vi "Project selector.vi"(11 "error in (no error)":errorcluster) -> (8 "OK":bool, 15 "error out":errorcluster)   [LabVIEW 2011]
doc: "Welcome screen, with basic options"
uses:
  GUI/Job setup/Job and site cluster.ctl
  emi cndiates/List of all contrys(combo box).ctl
  GUI/Job setup/Tool registration ID.ctl
  GUI/Job setup/Operators display clustor.ctl
  Application Structure/User Control/User Indikator.ctl
  Application Structure/User Control/Super User bool indikator.ctl
  Project infor with project path.ctl
  Project in icluster.ctl
  Run Information.ctl
panel:
  out "Comment":string
  in  "Project selector":u16(ring) items=["4325", "789"]
  in  "New project":bool
  in  "Operators":T1
  out "Tool":T2
  out "Job & Site":T3
  in  "Cancel":bool
  in  "OK btn":bool
  # "Comment"
  # "Tab header s can be changed as wanted\n\nCustom can be used for completly ccutom behavior,\nmust then highjack  an other hidden page, for settings"
  # "Add custom behavior taht cvan not be replicated by a simple cluster with valisdity checking"
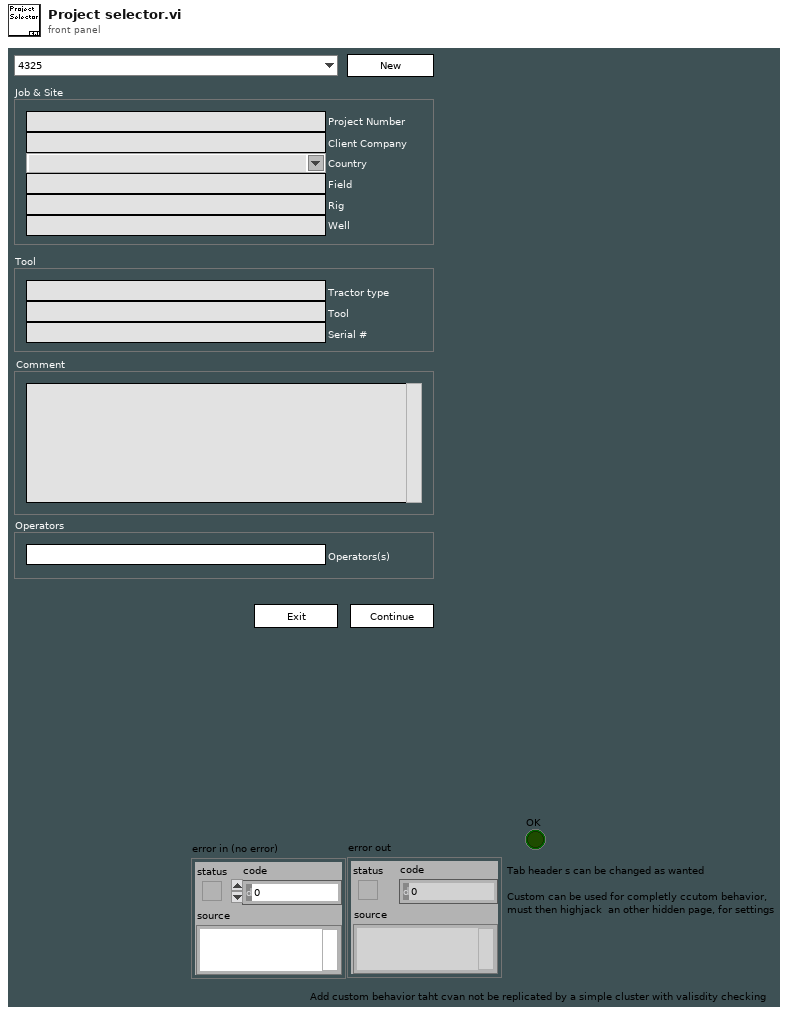
[diagram p1: front panel]
types:
  T1 = typedef "Operators display clustor.ctl" = cluster{"Operators(s)":string}
  T2 = typedef "Tool registration ID.ctl" = cluster{"Tractor type":string, "Tool":string, "Serial #":string}
  T3 = typedef "Job and site cluster.ctl" = cluster{"Project Number":string, "Client Company":string, "Country":T4, "Field":string, "Rig":string, "Well":string}
  T4 = typedef "List of all contrys(combo box).ctl" = string
  T5 = enum16{"GET", "SET", "Get from Ini", "Put in Ini"}
  T6 = typedef "User Indikator.ctl" = cluster{"User Name":string, "Super User":T7}
  T7 = typedef "Super User bool indikator.ctl" = bool
  T8 = typedef "Options  All pages and custom.ctl" = cluster{"P 1 (App)":T9, "P 2":T10, "P 3":T11, "P 4":T14, "P 5":T19, "P 6 (Err)":T20, "P 7 (Expert)":T21, "P 8 (Depth)":T23, "C 1":T24, "C 2":T25}
  T9 = typedef "Options Page 1 (App).ctl" = cluster{"Result files":path, "PCP Interface":string, "Tractor/Stroker Interface":string, "Tractor Interface":string, "Modem Status Interface":string, "Audible Alarm":bool, "Force alarm on Technical":bool, "Force alarm on HH":bool, "Force alarm on LL":bool, "Force alarm on H":bool, "Force alarm on L":bool}
  T10 = typedef "Options Page 2.ctl" = cluster{"Solenoid & Relay latching time":u16, "Tractor relay 1":dbl, "Tractor relay 2":dbl, "Tractor Solenoid limit":dbl}
  T11 = typedef "Options Page 3.ctl" = cluster{"Min resistance":dbl, "Max resistance":dbl, "Head voltage range":T12, "Max voltage jump":dbl, "Maximum resistance change":dbl, "Start Telemetry Voltage":dbl, "Start Telemetry Timeout":dbl, "Start Motor Voltage":dbl, "Stop Motor Voltage":dbl, "Pass Mode Warning Voltage":dbl, "Relay Switch Voltage":dbl, "Relay Status Loss Voltage":dbl, "Samples to average":i32, "PSU type DO NOT USE":T13, "Magna OVP":dbl, "Magna Current Limit":dbl}
  T12 = typedef "PCP type List.ctl" = enum16{"0 - 350V", "0 - 450V", "0 - 600V"}
  T13 = typedef "PSU Type.ctl" = enum16{"Unipower", "Magna 8.3A", "Magna 12A", "None"}
  T14 = typedef "Options Page 4.ctl" = cluster{"Solenoid & Relay latching time":u16, "Stroker relay 1":dbl, "Stroker Relay 2":dbl, "Stroker Solenoid limit":dbl, "Force det.":T15, "Stroke force lim.":dbl, "Anchor Enabled Pressure":dbl, "Tacometer puls":dbl, "Default anchor behavior":T16, "Default stroker behavior":T17, "Default stroker force limit (tonne)":dbl, "Slips Size":T18}
  T15 = typedef "Stroke force selector.ctl" = enum16{"Stroke in = node 1", "Strok out = node 1"}
  T16 = typedef "Default anchor behavior.ctl" = enum16{"Do nothing", "Set Anchor", "Release Anchor"}
  T17 = typedef "Default stroker behavior.ctl" = enum16{"Do nothing", "Stop", "Go Out", "Go In"}
  T18 = typedef "Slips Type Radio.ctl" = enum32{"No Selection", "338 MRS", "3,9 MRS"}
  T19 = typedef "Options Page 5.ctl" = cluster{"Solenoid & Relay latching time":u16, "Driller relay 1":dbl, "Driller Relay 2":dbl, "Driller  Solenoid limit":dbl}
  T20 = typedef "Options Page 6 (Err).ctl" = cluster{"Error and event files":path}
  T21 = typedef "Options Page 7 (Expert).ctl" = cluster{"Show Debug":bool, "Log debug messages":bool, "Additional debug messages":bool, "Start Beagle with Simulator data":bool, "Workshop mode":bool, "Modem baud":u16, "enumCANCOM":bool, "Modem sim":T22, "Telemetry Timeout Disable":i32, "Buffer size":i32, "Upd regular data":bool, "Cable comp":cluster{"VMOD1 Voltage(V)":dbl, "VMOD2 Voltage(V)":dbl}}
  T22 = typedef "Modem simulation setup.ctl" = cluster{"Modem dealay sim":bool, "Sim baud Tx":u16, "Bit Error fraction Tx":dbl, "Sim baud Rx":u16, "Bit Error fraction Rx":dbl}
  T23 = typedef "Options Page 8 (Depth).ctl" = cluster{"Winch Spool Circumference":dbl, "Winch Pulses per Revolution":dbl, "Current Depth":dbl}
  T24 = typedef "Options Custom 1.ctl" = cluster{"Depth Updated":bool, "Depth Offset":dbl}
  T25 = typedef "Options Custom 2.ctl" = cluster{"Placeholder":bool}
  T26 = typedef "Project infor with project path.ctl" = cluster{"Project path":path, "data":T27, "Comment":string}
  T27 = typedef "Project in icluster.ctl" = cluster{"Job and Site":T3, "Tool":T2, "Run Information":T28}
  T28 = typedef "Run Information.ctl" = cluster{"Active Run":bool, "String Check Rec":bool, "Run Number":i32, "Time of File Start":string}
  T29 = enum8{"Enabled", "Disabled", "Disabled and Grayed Out"}
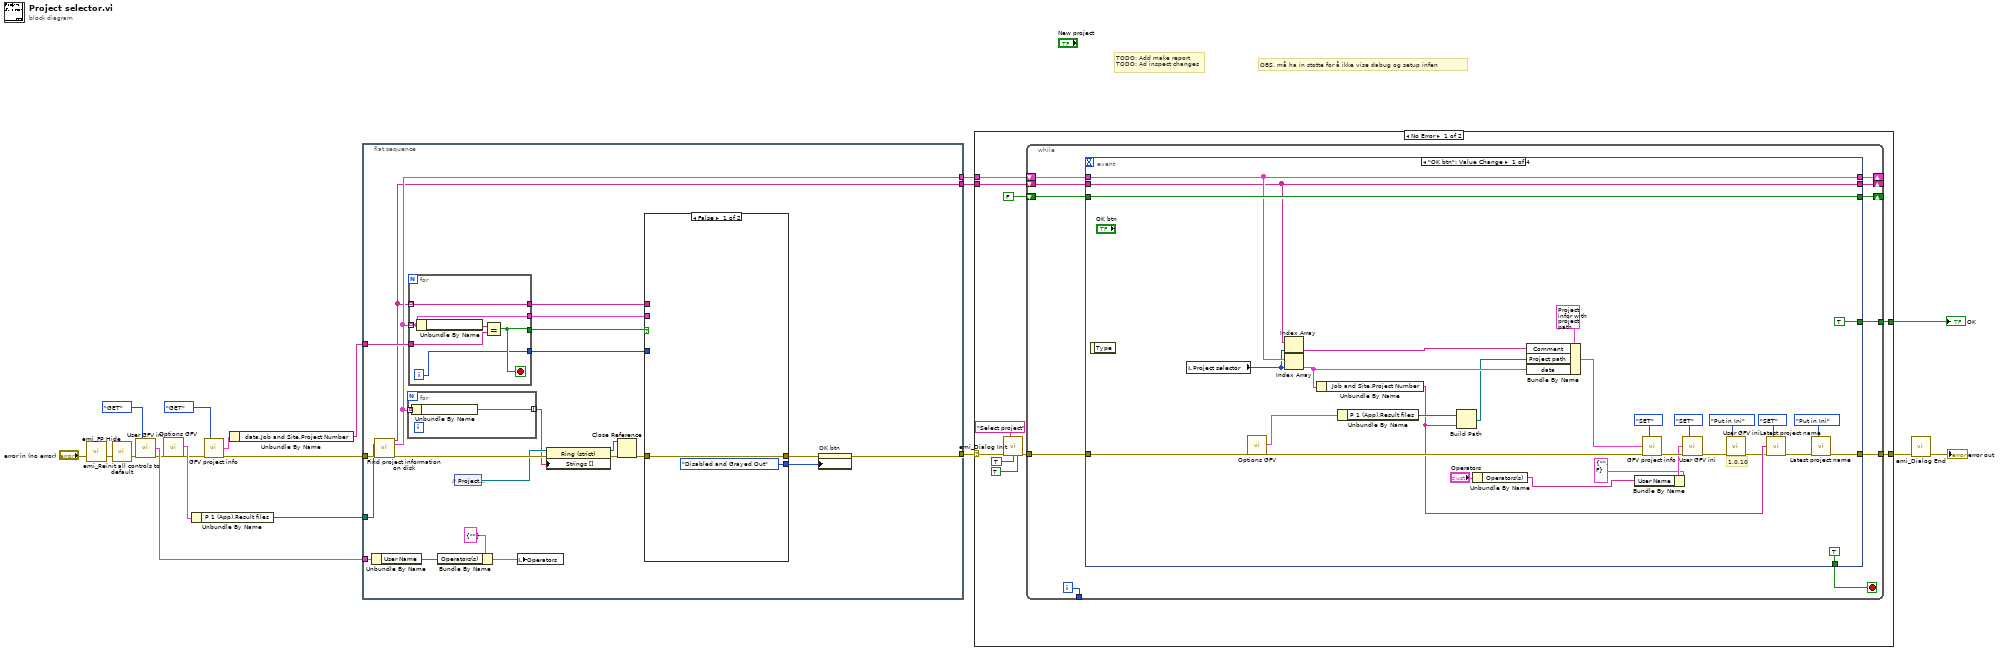
[diagram p0: block diagram]
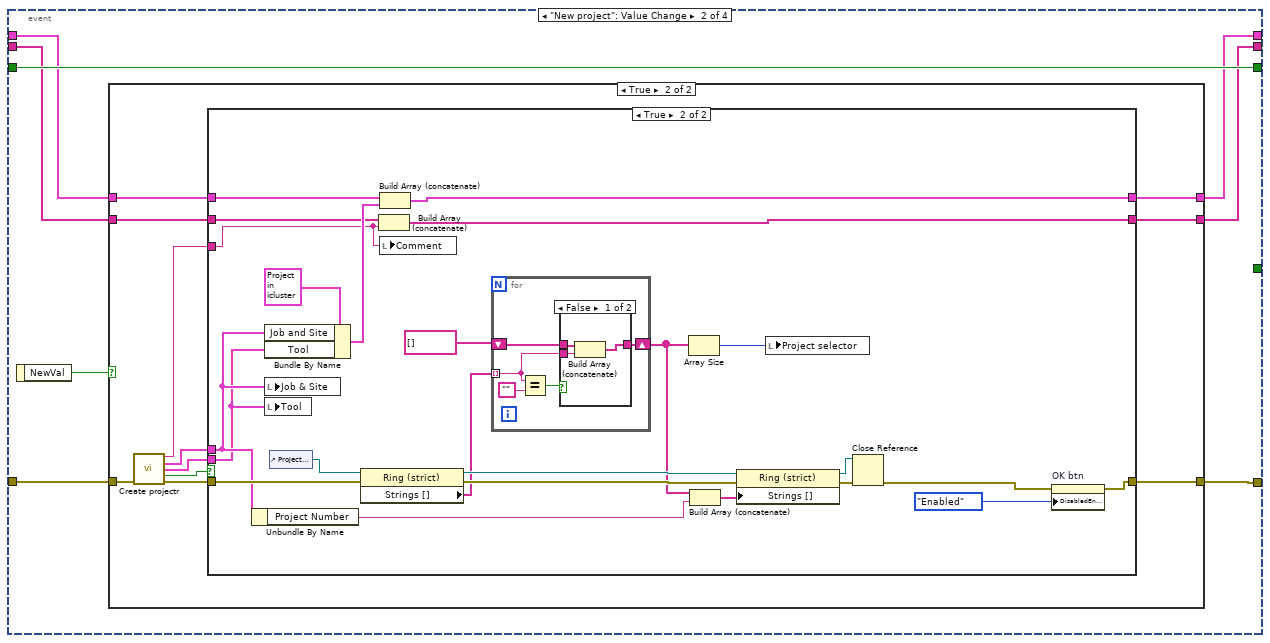
[diagram p2: hidden frame]
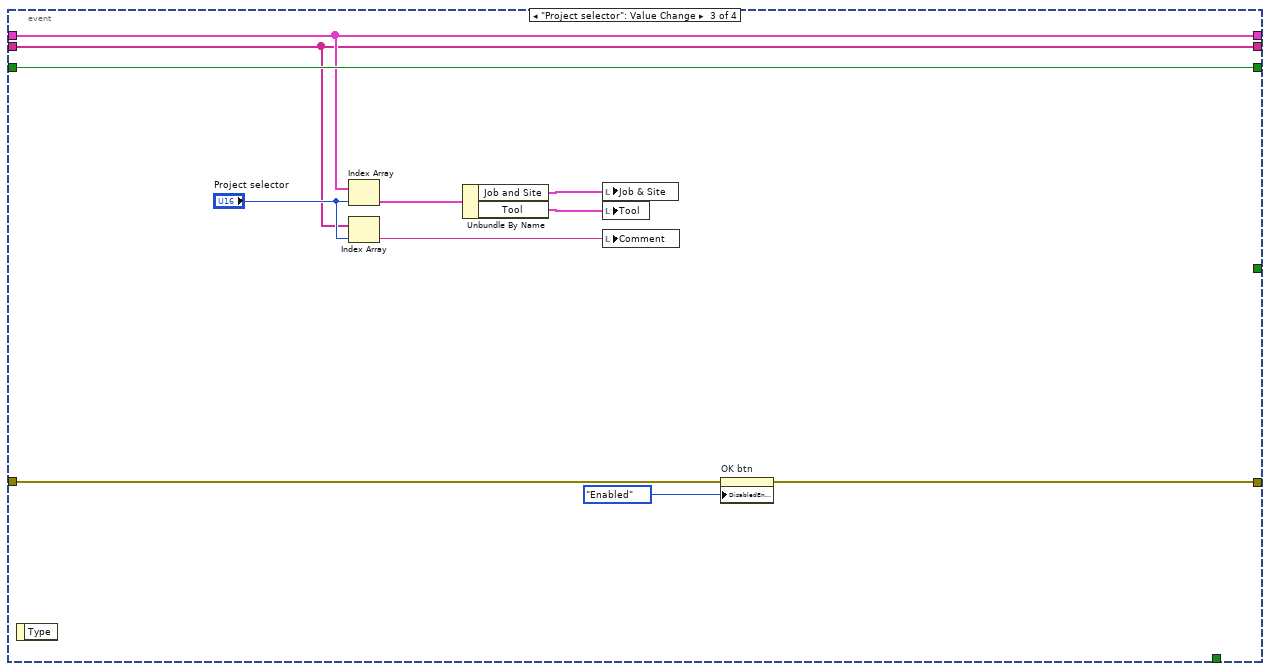
[diagram p6: hidden frame]
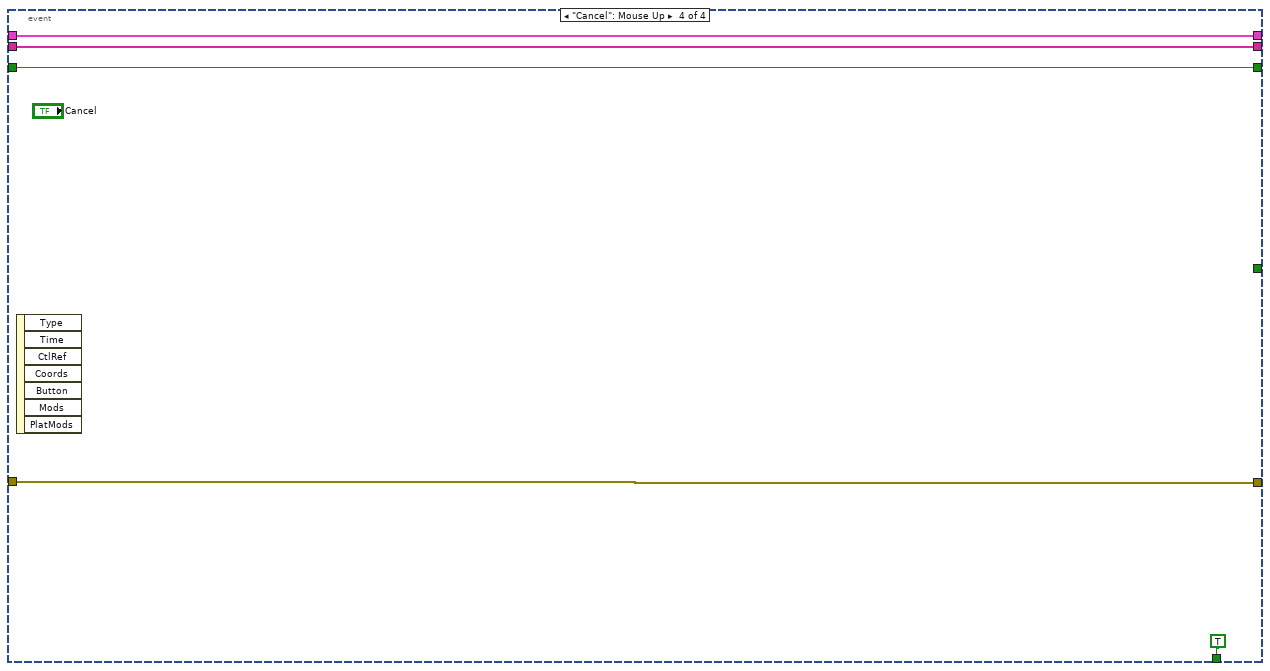
[diagram p7: hidden frame]
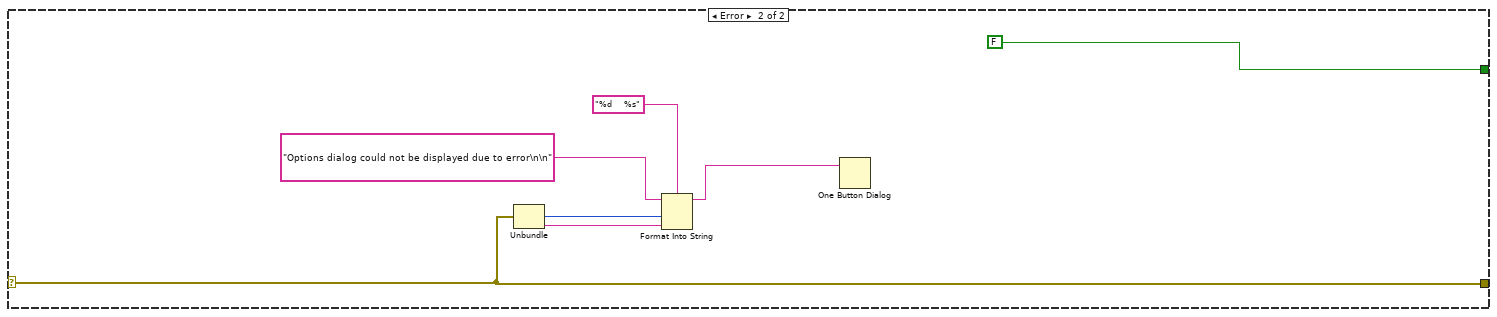
[diagram p8: hidden frame]
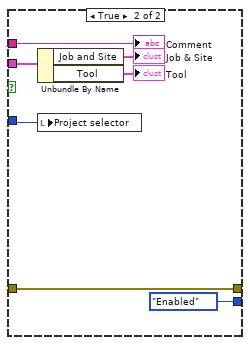
[diagram p9: hidden frame]
diagram:
  # "OBS, må ha in støtte for å ikke vise dabug og setup infen"
  # "TODO: Add make report\nTODO: Ad inspect changes"
  n1 = call "emi_FP Hide.vi"("error in (no error)"="error in (no error)") -> ("error out"=w15:errorcluster)  [unwired: 13 in, 1 out]
  n2 = call "emi_Reinit all controls to default.vi"("error in (no error)"=w15) -> ("error out"=w8:errorcluster)  [unwired: 13 in, 1 out]
  n3 = call "User GFV ini.vi"("Action(GET)"=T5."GET", "error in (no error)"=w8) -> ("User ID out"=w12:T6, "error out"=w11:errorcluster)  [unwired: 12 in]
  n4 = call "Options GFV.vi"("error in (no error)"=w11) -> ("Options"=w10:T8, "error out"=w6:errorcluster)  [unwired: 16 in, 1 out]
  n5 = Unbundle By Name(w10) -> ("P 1 (App).Result files"=w9:path)
  n6 = call "GFV project info.vi"("Action(GET)"=enum16{"GET", "SET"}."GET", "error in (no error)"=w6) -> ("Project info out"=w3:T26, "error out"=w5:errorcluster)  [unwired: 12 in]
  n7 = Unbundle By Name(w3) -> ("data.Job and Site.Project Number"=w2:string)
  n8 = flat-sequence {
    tunnel: [w25] -> w14
    tunnel: w5 -> [w41]
    tunnel: w12 -> [w21]
    tunnel: w9 -> [w40]
    tunnel: [w35] -> w7
    tunnel: w2 -> [w39]
    tunnel: [w27] -> w1
    frame #0 {
      n9 = Unbundle By Name(w21) -> ("User Name"=w20:string)
      n10 = call "Find project information on disk.vi"("Base folder"=w40, "error in (no error)"=w41) -> ("Comments"=w27:string[], "Project info"=w35:T27[], "error out"=w34:errorcluster)  [unwired: 10 in, 1 out]
      n11 = for {
        tunnel: w35 -> [w43] mode=indexing
        tunnel: [w42] -> w29 mode=indexing
        n12 = Unbundle By Name(w43) -> ("Job and Site.Project Number"=w42:string)
      }
      n13 = for {
        tunnel: w35 -> [w54] mode=indexing
        tunnel: w39 -> [w57]
        tunnel: [w56] -> w38
        tunnel: [w55] -> w36
        tunnel: [w54] -> w37
        tunnel: w27 -> [w53] mode=indexing
        tunnel: [w53] -> w28
        i -> [w55]
        stop <- w56 stop-if-true
        n14 = Unbundle By Name(w54) -> ("Job and Site.Project Number"=w58:string)
        n15 = Equal?(x=w58, y=w57) -> (x = y?=w56:bool)
      }
      n16 = Bundle By Name(cluster=T1 {"Operators(s)"=""} ("Operators"), "Operators(s)"=w20) -> (w22:T1)
      n17 = control-ref of="Project selector"() -> (w30:refnum<vi>)
      n18 = local write "Operators"(w22) -> ()
      n19 = property class="Ring (strict)"(reference=w30, error in=w34, "Strings []"=w29) -> (reference out=w31:refnum<vi>, error out=w33:errorcluster)
      n20 = Close Reference(reference=w31, error in (no error)=w33) -> (error out=w32:errorcluster)
      n21 = case shown="False" w38 {
        tunnel: [w45 w48] -> w26
        tunnel: w32 -> [w45 w48]
        tunnel: w37 -> [_ w51]
        tunnel: w36 -> [_ w52]
        tunnel: w28 -> [_ w47]
        tunnel: [T29."Disabled and Grayed Out" ("Disabled") T29."Enabled" ("Disabled")] -> w24
        frame False {
        }
        frame True {
          n22 = Unbundle By Name(w51) -> ("Job and Site"=→"Job & Site":T3, "Tool"=→"Tool":T2)
          n23 = local write "Project selector"(w52) -> ()
          "Comment" <- w47
        }
      }
      n24 = property on="OK btn" class="Bool (strict)"(error in=w26, "DisabledEnum"=w24) -> (error out=w25:errorcluster)  [unwired: 1 in, 1 out]
    }
  }
  n25 = case shown="No Error" w14 {
    selector: w14 -> [w63 w189]
    tunnel: [w68 FALSE] -> w18
    tunnel: [w67 w189] -> w17
    tunnel: w7 -> [w60 _]
    tunnel: w1 -> [w59 _]
    frame No Error {
      n26 = call "emi_Dialog Init.vi"("Header String(\"\")"="Select project" ("Header String(\"\")"), "error in"=w63, "Set BG Color(T)"=TRUE, "Modal(T)"=TRUE) -> ("error out"=w66:errorcluster)  [unwired: 11 in]
      n27 = while {
        tunnel: [w79] -> _
        tunnel: w66 -> [w77]
        tunnel: [w76] -> w67
        tunnel: [w75] -> w68
        shift-right: [w73] -> _
        shift-left: FALSE -> [w74]
        shift-right: [w71] -> _
        shift-left: w60 -> [w72]
        shift-right: [w69] -> _
        shift-left: w59 -> [w70]
        i -> [w79]
        stop <- w78 stop-if-true
        n28 = event shown="[0] \"OK btn\": Value Change" {
          selector: _ -> [_ _ _ _]
          dyn-events: _ -> [_ _ _ _]
          timeout: _ -> [_ _ _ _]
          tunnel: [TRUE _ _ TRUE] -> w78
          tunnel: w77 -> [w101 w115 w169 w182]
          tunnel: [w93 w114 w168 w182] -> w76
          tunnel: [TRUE _ _ _] -> w75
          tunnel: w74 -> [w108 w117 w178 w181]
          tunnel: [w108 w117 w178 w181] -> w73
          tunnel: w72 -> [w106 w113 w177 w180]
          tunnel: [w106 w112 w177 w180] -> w71
          tunnel: w70 -> [w88 w111 w172 w179]
          tunnel: [w88 w110 w172 w179] -> w69
          event "OK btn": Value Change {
            # "1.0.10"
            n29 = event-data() -> ()  [unwired: 1 in, 1 out]
            n30 = local read "Project selector"() -> (w89:u16)
            n31 = call "Options GFV.vi"("error in (no error)"=w101) -> ("Options"=w102:T8, "error out"=w100:errorcluster)  [unwired: 16 in, 1 out]
            n32 = Index Array(array=w88, index=w89) -> (element=w84:string)
            n33 = Index Array(array=w106, index=w89) -> (element=w98:T27)
            n34 = Unbundle By Name(w98) -> ("Job and Site.Project Number"=w92:string)
            n35 = Unbundle By Name(w102) -> ("P 1 (App).Result files"=w99:path)
            n36 = Build Path(base path=w99, name or relative path=w92) -> (appended path=w97:path)
            n37 = Unbundle By Name("Operators") -> ("Operators(s)"=w80:string)
            n38 = Bundle By Name(cluster=T26 {"Project path"=path "", "data"={"Job and Site"={"Project Number"="", "Client Company"="", "Country"="", "Field"="", "Rig"="", "Well"=""}, "Tool"={"Tractor type"="", "Tool"="", "Serial #"=""}, "Run Information"={"Active Run"=FALSE, "String Check Rec"=FALSE, "Run Number"=0, "Time of File Start"=""}}, "Comment"=""} ("Project info in"), "Comment"=w84, "Project path"=w97, "data"=w98) -> (w103:T26)
            n39 = Bundle By Name(cluster=T6 {"User Name"="", "Super User"=FALSE} ("User ID in"), "User Name"=w80) -> (w82:T6)
            n40 = call "GFV project info.vi"("Action(GET)"=enum16{"GET", "SET"}."SET", "Project info in"=w103, "error in (no error)"=w100) -> ("error out"=w96:errorcluster)  [unwired: 11 in, 1 out]
            n41 = call "User GFV ini.vi"("Action(GET)"=T5."SET", "User ID in"=w82, "error in (no error)"=w96) -> ("error out"=w87:errorcluster)  [unwired: 11 in, 1 out]
            n42 = call "User GFV ini.vi"("Action(GET)"=T5."Put in Ini", "error in (no error)"=w87) -> ("error out"=w85:errorcluster)  [unwired: 12 in, 1 out]
            n43 = call "Latest project name.vi"("Action(GET)"=T5."SET", "Project name"=w92, "error in (no error)"=w85) -> ("error out"=w94:errorcluster)  [unwired: 11 in, 1 out]
            n44 = call "Latest project name.vi"("Action(GET)"=T5."Put in Ini", "error in (no error)"=w94) -> ("error out"=w93:errorcluster)  [unwired: 12 in, 1 out]
          }
          event "New project": Value Change {
            n45 = event-data() -> ("NewVal"=w116:bool)  [unwired: 1 in]
            n46 = case shown="True" w116 {
              tunnel: w115 -> [w120 w131]
              tunnel: [w120 w130] -> w114
              tunnel: w113 -> [w119 w125]
              tunnel: [w119 w124] -> w112
              tunnel: w111 -> [w118 w122]
              tunnel: [w118 w121] -> w110
              frame False {
              }
              frame True {
                n47 = call "Create projectr.vi"("error in (no error)"=w131) -> ("Comment out"=w123:string, "Job & Site out"=w126:T3, "Tool out"=w127:T2, "OK"=w128:bool, "error out"=w129:errorcluster)  [unwired: 10 in]
                n48 = case shown="True" w128 {
                  tunnel: [w134 w135] -> w130
                  tunnel: w129 -> [w134 w153]
                  tunnel: w127 -> [_ w141]
                  tunnel: w126 -> [_ w142]
                  tunnel: w125 -> [w133 w158]
                  tunnel: [w133 w157] -> w124
                  tunnel: w123 -> [_ w138]
                  tunnel: w122 -> [w132 w140]
                  tunnel: [w132 w139] -> w121
                  frame False {
                  }
                  frame True {
                    n49 = Unbundle By Name(w142) -> ("Project Number"=w148:string)
                    n50 = Bundle By Name(cluster=T27 {"Job and Site"={"Project Number"="", "Client Company"="", "Country"="", "Field"="", "Rig"="", "Well"=""}, "Tool"={"Tractor type"="", "Tool"="", "Serial #"=""}, "Run Information"={"Active Run"=FALSE, "String Check Rec"=FALSE, "Run Number"=0, "Time of File Start"=""}} ("Project information"), "Job and Site"=w142, "Tool"=w141) -> (w155:T27)
                    n51 = local write "Job & Site"(w142) -> ()
                    n52 = local write "Tool"(w141) -> ()
                    n53 = control-ref of="Project selector"() -> (w154:refnum<vi>)
                    n54 = property class="Ring (strict)"(reference=w154, error in=w153) -> (reference out=w151:refnum<vi>, error out=w152:errorcluster, "Strings []"=w145:string[])
                    n55 = Build Array (concatenate)(w140, w138) -> (w139:string[])
                    n56 = Build Array (concatenate)(w158, w155) -> (w157:T27[])
                    n57 = local write "Comment"(w138) -> ()
                    n58 = for {
                      tunnel: w145 -> [w159] mode=indexing
                      shift-right: [w161] -> w143
                      shift-left: string[] [] ("Strings []") -> [w160]
                      n59 = Equal?(x=w159, y="") -> (x = y?=w162:bool)
                      n60 = case shown="False" w162 {
                        tunnel: [w165 w167] -> w161
                        tunnel: w160 -> [w166 w167]
                        tunnel: w159 -> [w164 _]
                        frame False {
                          n61 = Build Array (concatenate)(w166, w164) -> (w165:string[])
                        }
                        frame True {
                        }
                      }
                    }
                    n62 = Array Size(array=w143) -> (size(s)=w146:i32)
                    n63 = Build Array (concatenate)(w143, w148) -> (w147:string[])
                    n64 = property class="Ring (strict)"(reference=w151, error in=w152, "Strings []"=w147) -> (reference out=w149:refnum<vi>, error out=w150:errorcluster)
                    n65 = local write "Project selector"(w146) -> ()
                    n66 = Close Reference(reference=w149, error in (no error)=w150) -> (error out=w136:errorcluster)
                    n67 = property on="OK btn" class="Bool (strict)"(error in=w136, "DisabledEnum"=T29."Enabled" ("Disabled")) -> (error out=w135:errorcluster)  [unwired: 1 in, 1 out]
                  }
                }
              }
            }
          }
          event "Project selector": Value Change {
            n68 = event-data() -> ()  [unwired: 1 in, 1 out]
            n69 = Index Array(array=w177, index="Project selector") -> (element=w176:T27)
            n70 = Index Array(array=w172, index="Project selector") -> (element=w171:string)
            n71 = Unbundle By Name(w176) -> ("Job and Site"=w175:T3, "Tool"=w174:T2)
            n72 = local write "Job & Site"(w175) -> ()
            n73 = local write "Tool"(w174) -> ()
            n74 = local write "Comment"(w171) -> ()
            n75 = property on="OK btn" class="Bool (strict)"(error in=w169, "DisabledEnum"=T29."Enabled" ("Disabled")) -> (error out=w168:errorcluster)  [unwired: 1 in, 1 out]
          }
          event "Cancel": Mouse Up {
            n76 = event-data() -> ()  [unwired: 1 in, 7 out]
          }
        }
      }
    }
    frame Error {
      n77 = Unbundle(w189) -> ("code"=w186:i32, "source"=w185:string)  [unwired: 1 out]
      n78 = Format Into String(format string="%d    %s", initial string="Options dialog could not be displayed due to error\n\n" ("message"), w186, w185) -> (resulting string=w187:string)  [unwired: 1 in, 1 out]
      n79 = One Button Dialog(message=w187) -> ()  [unwired: 1 in, 1 out]
    }
  }
  "OK" <- w18
  n80 = call "emi_Dialog End.vi"("error in"=w17) -> ("error out"=→"error out":errorcluster)  [unwired: 14 in]
